vi "Flatten To String.vi"(8 "error in (no error)":errorcluster, 10 "Variant":variant, 11 "JSON Serializer in":refnum<class "JSON Serializer.lvclass">) -> (0 "error out":errorcluster, 2 "String":string, 3 "JSON Serializer out":refnum<class "JSON Serializer.lvclass">)   [LabVIEW 2017, in "JKI JSON Serialization.lvlib" / "JSON Serializer.lvclass"]
doc: "Converts <b>Variant</b> to JSON formatted <b>String</b>."
uses:
  JSON Serializer.lvclass
  JSON Serializer.lvclass/JSON Serializer.ctl
  <vilib>/Utility/error.llb/whitespace.ctl
  <vilib>/Utility/VariantDataType/VariantType.lvlib
  JKI JSON Serialization.lvlib
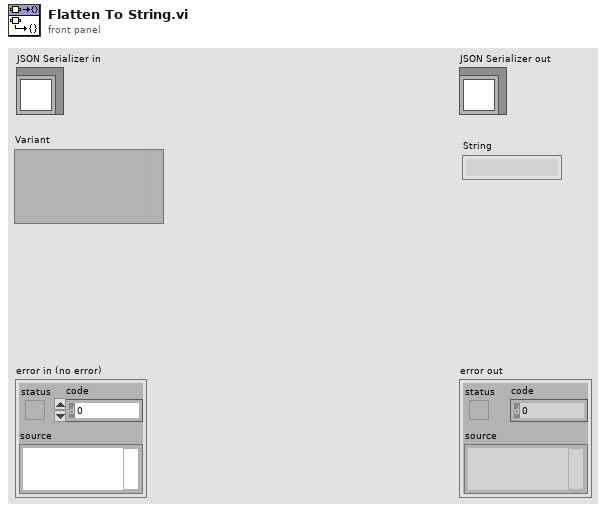
[diagram p1: front panel]
types:
  T1 = typedef "VariantType.lvlib/Type.ctl" = enum8{"Invalid Type", "Void", "I8", "I16", "I32", "I64", "U8", "U16", "U32", "U64", "Single Float", "Double Float", "Extended Float", "Single Complex", "Double Complex", "Extended Complex", "Enum U8", "Enum U16", "Enum U32", "Enum U64", "Single Float With Unit", "Double Float With Unit", "Extended Float With Unit", "Single Complex with Unit", "Double Complex with Unit", "Extended Complex with Unit", "Boolean", "String", "Path", "Picture", "Tag", "Array", "Cluster", "Variant", "LV Variant", "Waveform", "Timestamp", "Digital Waveform", "Digital Data", "ExpressData", "Refnum", "External Data", "VI", "Poly VI", "LabVIEW Class Instance", "Fixed Point"}
  T2 = typedef "whitespace.ctl" = u16
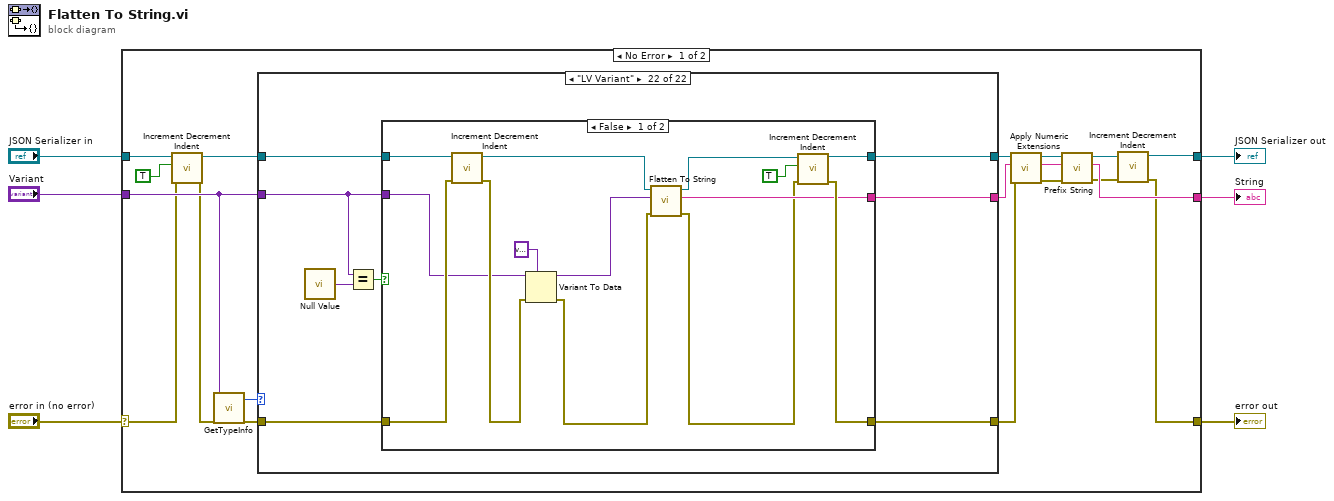
[diagram p0: block diagram]
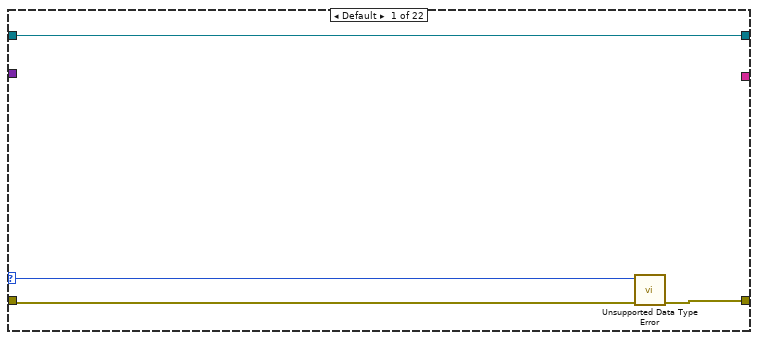
[diagram p2: hidden frame]
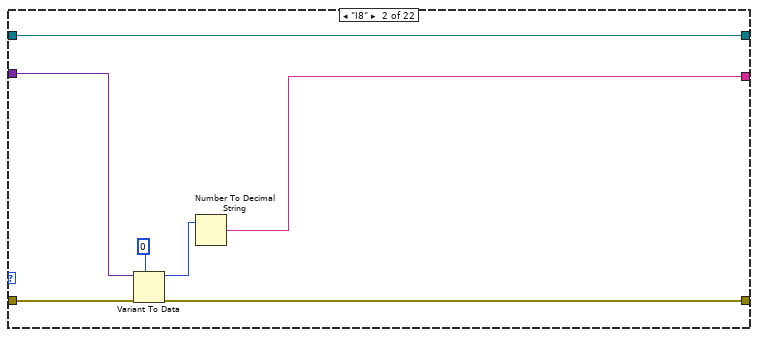
[diagram p3: hidden frame]
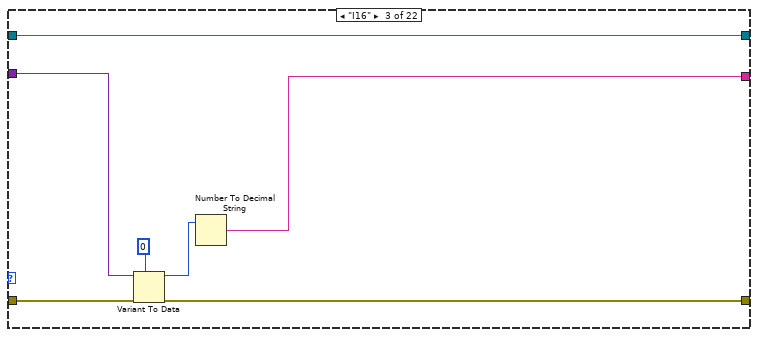
[diagram p4: hidden frame]
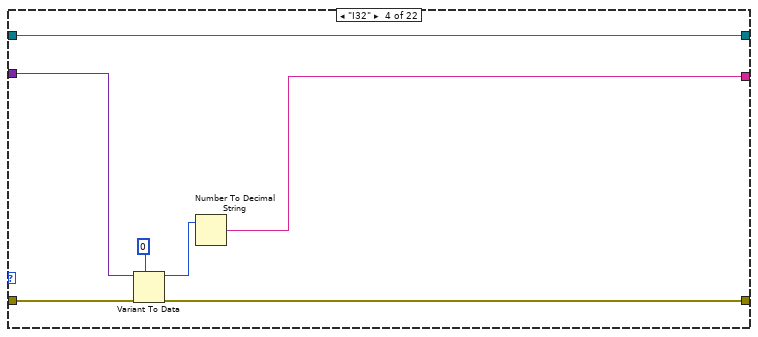
[diagram p5: hidden frame]
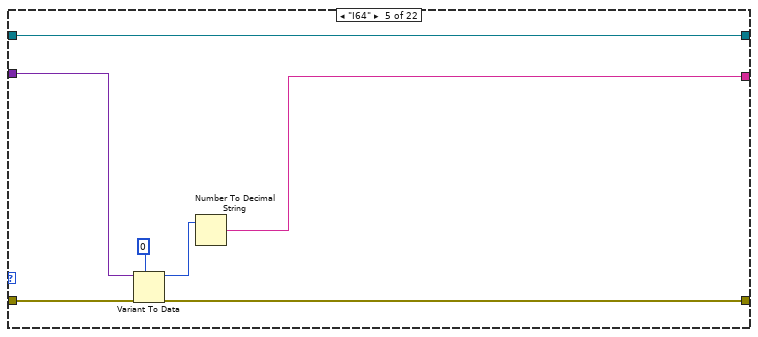
[diagram p6: hidden frame]
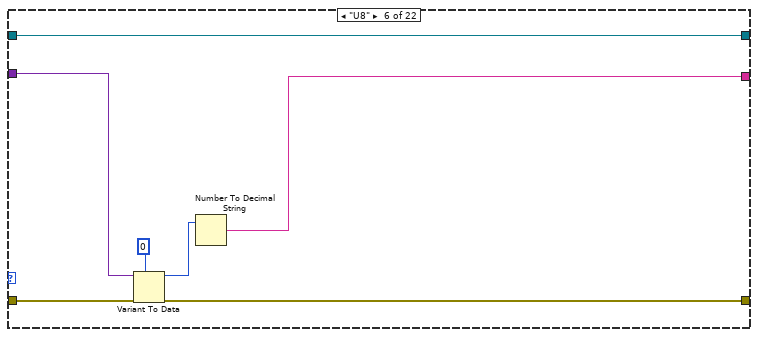
[diagram p7: hidden frame]
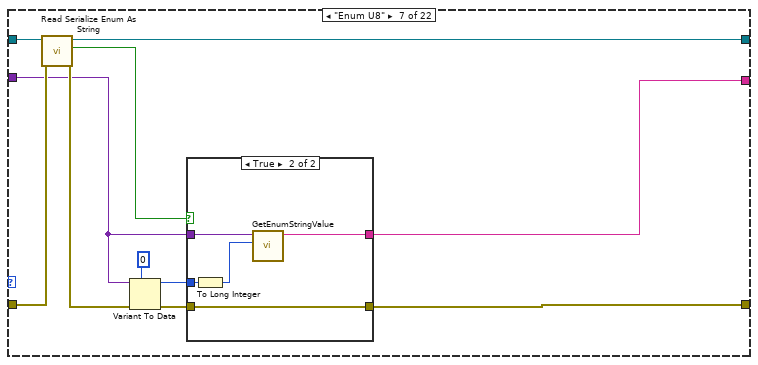
[diagram p8: hidden frame]
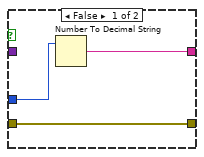
[diagram p9: hidden frame]
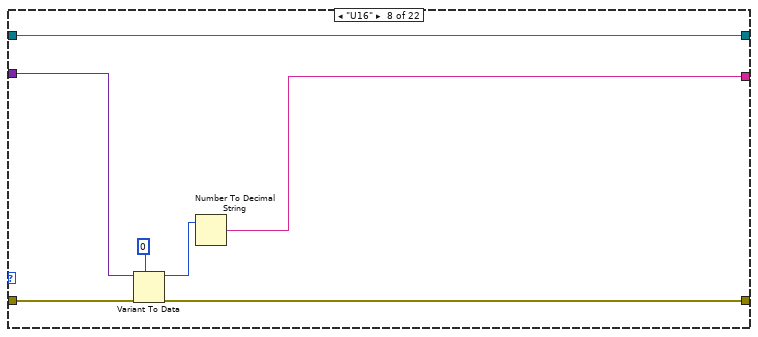
[diagram p10: hidden frame]
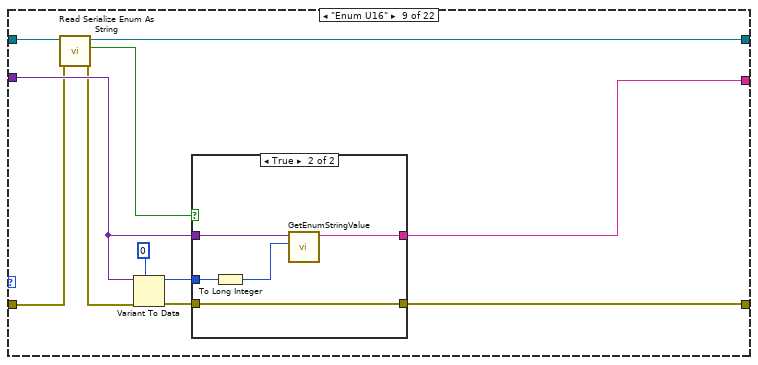
[diagram p11: hidden frame]
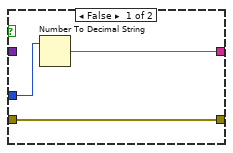
[diagram p12: hidden frame]
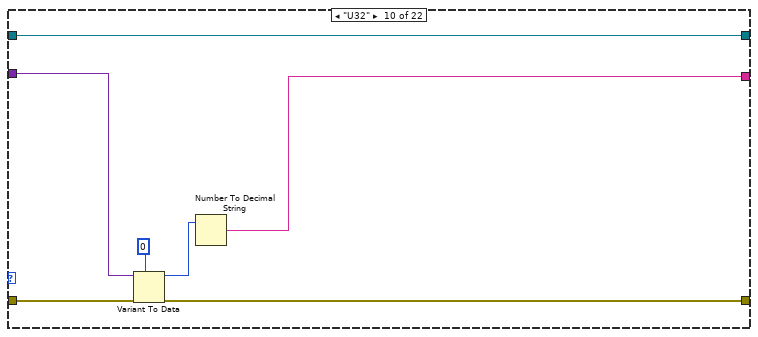
[diagram p13: hidden frame]
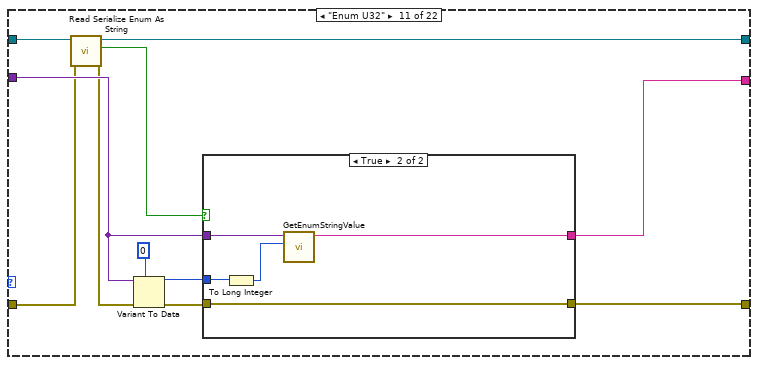
[diagram p14: hidden frame]
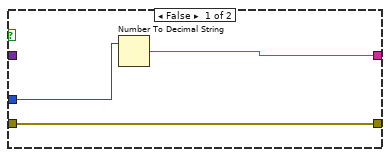
[diagram p15: hidden frame]
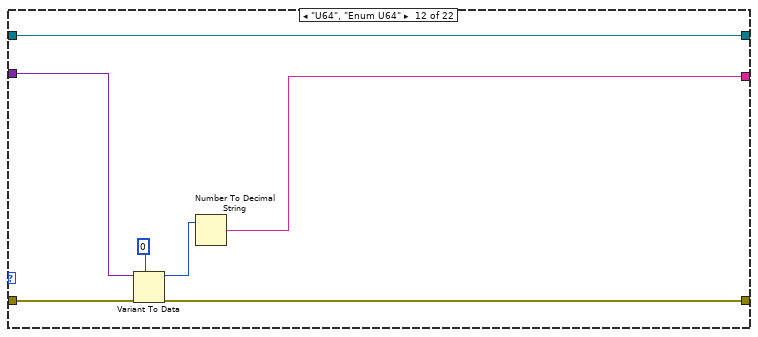
[diagram p16: hidden frame]
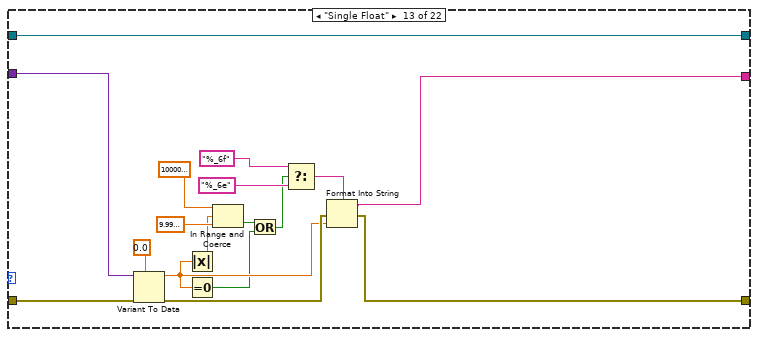
[diagram p17: hidden frame]
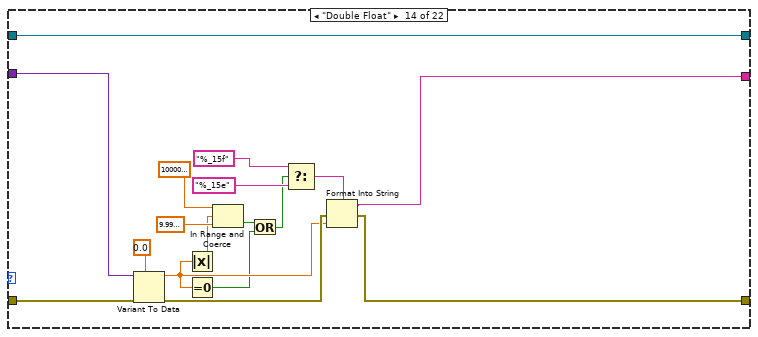
[diagram p18: hidden frame]
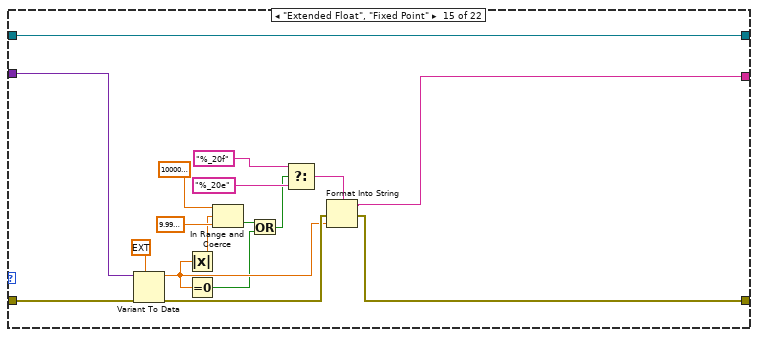
[diagram p19: hidden frame]
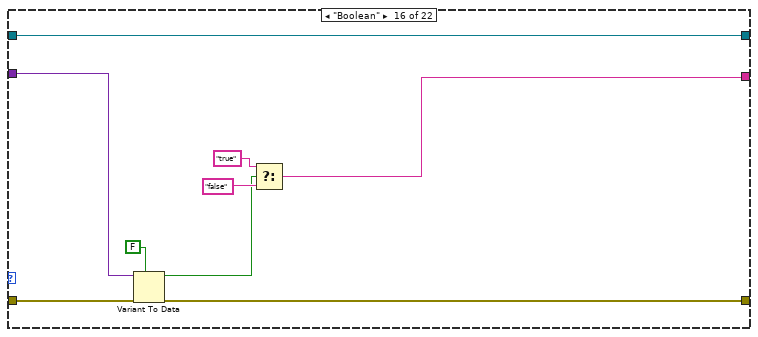
[diagram p20: hidden frame]
diagram:
  n1 = case shown="No Error" "error in (no error)" {
    selector: "error in (no error)" -> [w18 w436]
    tunnel: [w7 w436] -> w5
    tunnel: [w9 w435] -> w3
    tunnel: "JSON Serializer in" -> [w20 w435]
    tunnel: "Variant" -> [w23 _]
    tunnel: [w12 _] -> w1
    frame No Error {
      n2 = call "Increment Decrement Indent.vi"("error in (no error)"=w18, "Increment"=TRUE, "JSON Serializer in"=w20) -> ("error out"=w17:errorcluster, "JSON Serializer out"=w19:refnum<class "JSON Serializer.lvclass">)  [unwired: 7 in]
      n3 = call <vilib>:"GetTypeInfo.vi"("error in (no error)"=w17, "Variant"=w23) -> ("error out"=w24:errorcluster, "Type Enum"=w25:T1)  [unwired: 5 in, 3 out]
      n4 = case shown="\"LV Variant\"" w25 {
        selector: w25 -> [w26 _ _ _ _ _ _ _ _ _ _ _ _ _ _ _ w203 w250 _ _ _ _]
        tunnel: w19 -> [w29 w36 w43 w50 w57 w64 w74 w90 w95 w116 w125 w142 w159 w176 w193 w202 w208 w248 w275 w323 w358 w414]
        tunnel: [w29 w36 w43 w50 w57 w64 w73 w90 w94 w116 w124 w142 w159 w176 w193 w202 w208 w247 w274 w321 w361 w417] -> w15
        tunnel: [w28 w30 w37 w44 w51 w58 w65 w84 w98 w110 w122 w136 w154 w171 w188 w194 w205 w251 w273 w320 w360 w416] -> w22
        tunnel: w24 -> [w27 w35 w42 w49 w56 w63 w72 w89 w93 w115 w118 w141 w158 w175 w192 w201 w207 w249 w271 w324 w362 w413]
        tunnel: [_ w31 w38 w45 w52 w59 w75 w85 w97 w111 w123 w137 w148 w165 w182 w196 w204 w245 w272 w319 w359 w415] -> w21
        tunnel: w23 -> [_ w34 w41 w48 w55 w62 w67 w88 w96 w114 w119 w140 w157 w174 w191 w200 w206 w243 w269 w322 w363 w411]
        frame Default {
          n5 = call "Unsupported Data Type Error.vi"("error in (no error)"=w27, "Type Enum"=w26) -> ("error out"=w28:errorcluster)  [unwired: 9 in]
        }
        frame "I8" {
          n6 = Variant To Data(error in=w35, type=i8 0, Variant=w34) -> (data=w32:i8, error out=w30:errorcluster)
          n7 = Number To Decimal String(number=w32) -> (decimal integer string=w31:string)  [unwired: 1 in]
        }
        frame "I16" {
          n8 = Variant To Data(error in=w42, type=i16 0, Variant=w41) -> (data=w39:i16, error out=w37:errorcluster)
          n9 = Number To Decimal String(number=w39) -> (decimal integer string=w38:string)  [unwired: 1 in]
        }
        frame "I32" {
          n10 = Variant To Data(error in=w49, type=0, Variant=w48) -> (data=w46:i32, error out=w44:errorcluster)
          n11 = Number To Decimal String(number=w46) -> (decimal integer string=w45:string)  [unwired: 1 in]
        }
        frame "I64" {
          n12 = Variant To Data(error in=w56, type=i64 0, Variant=w55) -> (data=w53:i64, error out=w51:errorcluster)
          n13 = Number To Decimal String(number=w53) -> (decimal integer string=w52:string)  [unwired: 1 in]
        }
        frame "U8" {
          n14 = Variant To Data(error in=w63, type=u8 0, Variant=w62) -> (data=w60:u8, error out=w58:errorcluster)
          n15 = Number To Decimal String(number=w60) -> (decimal integer string=w59:string)  [unwired: 1 in]
        }
        frame "Enum U8" {
          n16 = call-dynamic "Read Serialize Enum As String.vi"("error in (no error)"=w72, "JSON Serializer in"=w74) -> ("error out"=w71:errorcluster, "Enums As String?"=w68:bool, "JSON Serializer out"=w73:refnum<class "JSON Serializer.lvclass">)  [unwired: 7 in]
          n17 = Variant To Data(error in=w71, type=u8 0, Variant=w67) -> (data=w69:u8, error out=w66:errorcluster)
          n18 = case shown="True" w68 {
            tunnel: [w78 w79] -> w75
            tunnel: w69 -> [w77 w81]
            tunnel: w67 -> [_ w82]
            tunnel: w66 -> [w76 w83]
            tunnel: [w76 w83] -> w65
            frame False {
              n19 = Number To Decimal String(number=w77) -> (decimal integer string=w78:string)  [unwired: 1 in]
            }
            frame True {
              n20 = To Long Integer(number=w81) -> (32bit integer=w80:i32)
              n21 = call "GetEnumStringValue.vi"("Index"=w80, "Enum Variant"=w82) -> ("string"=w79:string)  [unwired: 9 in]
            }
          }
        }
        frame "U16" {
          n22 = Variant To Data(error in=w89, type=u16 0, Variant=w88) -> (data=w86:u16, error out=w84:errorcluster)
          n23 = Number To Decimal String(number=w86) -> (decimal integer string=w85:string)  [unwired: 1 in]
        }
        frame "Enum U16" {
          n24 = call-dynamic "Read Serialize Enum As String.vi"("error in (no error)"=w93, "JSON Serializer in"=w95) -> ("error out"=w92:errorcluster, "Enums As String?"=w91:bool, "JSON Serializer out"=w94:refnum<class "JSON Serializer.lvclass">)  [unwired: 7 in]
          n25 = Variant To Data(error in=w92, type=u16 0, Variant=w96) -> (data=w100:u16, error out=w99:errorcluster)
          n26 = case shown="True" w91 {
            tunnel: [w104 w105] -> w97
            tunnel: w100 -> [w103 w107]
            tunnel: w96 -> [_ w108]
            tunnel: w99 -> [w102 w106]
            tunnel: [w102 w106] -> w98
            frame False {
              n27 = Number To Decimal String(number=w103) -> (decimal integer string=w104:string)  [unwired: 1 in]
            }
            frame True {
              n28 = To Long Integer(number=w107) -> (32bit integer=w109:i32)
              n29 = call "GetEnumStringValue.vi"("Index"=w109, "Enum Variant"=w108) -> ("string"=w105:string)  [unwired: 9 in]
            }
          }
        }
        frame "U32" {
          n30 = Variant To Data(error in=w115, type=u32 0, Variant=w114) -> (data=w112:u32, error out=w110:errorcluster)
          n31 = Number To Decimal String(number=w112) -> (decimal integer string=w111:string)  [unwired: 1 in]
        }
        frame "Enum U32" {
          n32 = call-dynamic "Read Serialize Enum As String.vi"("error in (no error)"=w118, "JSON Serializer in"=w125) -> ("error out"=w117:errorcluster, "Enums As String?"=w126:bool, "JSON Serializer out"=w124:refnum<class "JSON Serializer.lvclass">)  [unwired: 7 in]
          n33 = Variant To Data(error in=w117, type=u32 0, Variant=w119) -> (data=w120:u32, error out=w121:errorcluster)
          n34 = case shown="True" w126 {
            tunnel: [w130 w131] -> w123
            tunnel: w120 -> [w129 w132]
            tunnel: w119 -> [_ w133]
            tunnel: w121 -> [w128 w135]
            tunnel: [w128 w135] -> w122
            frame False {
              n35 = Number To Decimal String(number=w129) -> (decimal integer string=w130:string)  [unwired: 1 in]
            }
            frame True {
              n36 = To Long Integer(number=w132) -> (32bit integer=w134:i32)
              n37 = call "GetEnumStringValue.vi"("Index"=w134, "Enum Variant"=w133) -> ("string"=w131:string)  [unwired: 9 in]
            }
          }
        }
        frame "U64", "Enum U64" {
          n38 = Variant To Data(error in=w141, type=u64 0, Variant=w140) -> (data=w138:u64, error out=w136:errorcluster)
          n39 = Number To Decimal String(number=w138) -> (decimal integer string=w137:string)  [unwired: 1 in]
        }
        frame "Single Float" {
          n40 = Variant To Data(error in=w158, type=sgl 0.0, Variant=w157) -> (data=w146:sgl, error out=w155:errorcluster)
          n41 = Absolute Value(x=w146) -> (abs(x)=w147:sgl)
          n42 = Equal To 0?(x=w146) -> (x = 0?=w145:bool)
          n43 = In Range and Coerce(upper limit=sgl 1000000.0, x=w147, lower limit=sgl 0.0001 ("upper limit")) -> (In Range?=w144:bool)  [unwired: 1 out]
          n44 = Or(x=w144, y=w145) -> (x .or. y?=w143:bool)
          n45 = Select(t="%_6f" ("format string"), s=w143, f="%_6e" ("format string")) -> (s? t:f=w149:string)
          n46 = Format Into String(format string=w149, error in=w155, w146) -> (resulting string=w148:string, error out=w154:errorcluster)  [unwired: 1 in]
        }
        frame "Double Float" {
          n47 = Variant To Data(error in=w175, type=0.0, Variant=w174) -> (data=w163:dbl, error out=w172:errorcluster)
          n48 = Absolute Value(x=w163) -> (abs(x)=w164:dbl)
          n49 = Equal To 0?(x=w163) -> (x = 0?=w162:bool)
          n50 = In Range and Coerce(upper limit=sgl 1000000.0, x=w164, lower limit=sgl 0.0001 ("upper limit")) -> (In Range?=w161:bool)  [unwired: 1 out]
          n51 = Or(x=w161, y=w162) -> (x .or. y?=w160:bool)
          n52 = Select(t="%_15f" ("format string"), s=w160, f="%_15e" ("format string")) -> (s? t:f=w166:string)
          n53 = Format Into String(format string=w166, error in=w172, w163) -> (resulting string=w165:string, error out=w171:errorcluster)  [unwired: 1 in]
        }
        frame "Extended Float", "Fixed Point" {
          n54 = Variant To Data(error in=w192, type=ext 0.0, Variant=w191) -> (data=w180:ext, error out=w189:errorcluster)
          n55 = Absolute Value(x=w180) -> (abs(x)=w181:ext)
          n56 = Equal To 0?(x=w180) -> (x = 0?=w179:bool)
          n57 = In Range and Coerce(upper limit=sgl 1000000.0, x=w181, lower limit=sgl 0.0001 ("upper limit")) -> (In Range?=w178:bool)  [unwired: 1 out]
          n58 = Or(x=w178, y=w179) -> (x .or. y?=w177:bool)
          n59 = Select(t="%_20f" ("format string"), s=w177, f="%_20e" ("format string")) -> (s? t:f=w183:string)
          n60 = Format Into String(format string=w183, error in=w189, w180) -> (resulting string=w182:string, error out=w188:errorcluster)  [unwired: 1 in]
        }
        frame "Boolean" {
          n61 = Variant To Data(error in=w201, type=FALSE, Variant=w200) -> (data=w195:bool, error out=w194:errorcluster)
          n62 = Select(t="true" ("format string"), s=w195, f="false" ("format string")) -> (s? t:f=w196:string)
        }
        frame "String", "Path" {
          n63 = case shown="\"Path\"" w203 {
            tunnel: w207 -> [w216 w242]
            tunnel: w206 -> [w215 w241]
            tunnel: [w214 w237] -> w205
            tunnel: [w213 w231] -> w204
            frame "Path" {
              n64 = Variant To Data(error in=w216, type=path "", Variant=w215) -> (data=w209:path, error out=w211:errorcluster)
              n65 = Not A Number/Path/Refnum?(number/path/refnum=w209) -> (NaN/Path/Refnum?=w210:bool)
              n66 = case shown="True" w210 {
                tunnel: [w225 w229] -> w214
                tunnel: [w219 "null" ("JSON string")] -> w213
                tunnel: w211 -> [w217 w229]
                tunnel: w209 -> [w218 _]
                frame False {
                  n67 = Path To String(path=w218) -> (string=w226:string)
                  n68 = Build Array(w226) -> (w227:string[])
                  n69 = Flatten To JSON(anything=w227, error in (no error)=w217) -> (JSON string=w223:string, 11:w225:errorcluster)  [unwired: 1 in]
                  n70 = String Length(string=w223) -> (length=w222:i32)
                  n71 = Subtract(x=w222, y=2) -> (x-y=w220:i32)
                  n72 = String Subset(string=w223, offset (0)=1, length (rest)=w220) -> (substring=w219:string)
                }
                frame True {
                }
              }
            }
            frame "String", Default {
              n73 = Variant To Data(error in=w242, type="", Variant=w241) -> (data=w239:string, error out=w238:errorcluster)
              n74 = Build Array(w239) -> (w240:string[])
              n75 = Flatten To JSON(anything=w240, error in (no error)=w238) -> (JSON string=w235:string, 11:w237:errorcluster)  [unwired: 1 in]
              n76 = String Length(string=w235) -> (length=w234:i32)
              n77 = Subtract(x=w234, y=2) -> (x-y=w232:i32)
              n78 = String Subset(string=w235, offset (0)=1, length (rest)=w232) -> (substring=w231:string)
            }
          }
        }
        frame "Timestamp" {
          n79 = Unbundle By Name(w248) -> ("timestamps"=w246:bool, "universal time"=w244:bool)
          n80 = case shown="True" w246 {
            tunnel: [w255 w256] -> w251
            tunnel: w250 -> [w254 _]
            tunnel: w249 -> [w253 w266]
            tunnel: w248 -> [w252 w267]
            tunnel: [w252 w267] -> w247
            tunnel: [_ w258] -> w245
            tunnel: w244 -> [_ w261]
            tunnel: w243 -> [_ w265]
            frame False {
              n81 = call "Unsupported Data Type Error.vi"("error in (no error)"=w253, "Type Enum"=w254) -> ("error out"=w255:errorcluster)  [unwired: 9 in]
            }
            frame True {
              n82 = Variant To Data(error in=w266, type=timestamp(0 s since 1904-01-01), Variant=w265) -> (data=w264:timestamp, error out=w262:errorcluster)
              n83 = call "Timestamp To ISO String.vi"("error in (no error)"=w262, "Universal time (F)"=w261, "Timestamp"=w264) -> ("error out"=w257:errorcluster, "ISO Timestamp String"=w259:string)  [unwired: 7 in]
              n84 = Format Into String(format string="\"%s\"", error in=w257, w259) -> (resulting string=w258:string, error out=w256:errorcluster)  [unwired: 1 in]
            }
          }
        }
        frame "Array" {
          n85 = call <vilib>:"GetArrayInfo.vi"("error in (no error)"=w271, "Variant"=w269) -> ("error out"=w270:errorcluster, "NDims"=w268:i32)  [unwired: 6 in, 2 out]
          n86 = case shown="2.." w268 {
            tunnel: w275 -> [w276 w292 w312]
            tunnel: [w276 w289 w310] -> w274
            tunnel: [w279 w287 w308] -> w273
            tunnel: [_ w286 w307] -> w272
            tunnel: w270 -> [w277 w282 w302]
            tunnel: w269 -> [_ w281 w303]
            frame 0, Default {
              n87 = call <vilib>:"Error Cluster From Error Code.vi"("error in (no error)"=w277, "error message (\"\")"="Flattening failed. Zero or negative dimensional arrays not supported." ("error message (\"\")"), "error code (0)"=1) -> ("error out"=w279:errorcluster)  [unwired: 6 in]
            }
            frame 1 {
              n88 = call <userlib>:"Array to Array of VData__ogtk.vi"("error in (no error)"=w282, "MultiD Array"=w281) -> ("error out"=w291:errorcluster, "1D Array of Variants"=w293:variant[])  [unwired: 8 in]
              n89 = for {
                tunnel: w293 -> [w299] mode=indexing
                shift-right: [w297] -> w290
                shift-left: w292 -> [w298]
                tunnel: [w296] -> w285 mode=indexing
                shift-right: [w295] -> w288
                shift-left: w291 -> [w294]
                n90 = call-dynamic "Flatten To String.vi"("error in (no error)"=w294, "Variant"=w299, "JSON Serializer in"=w298) -> ("error out"=w295:errorcluster, "String"=w296:string, "JSON Serializer out"=w297:refnum<class "JSON Serializer.lvclass">)  [unwired: 6 in]
              }
              n91 = call "Prefix Array.vi"("End Symbol"="]", "Start Symbol"="[", "error in (no error)"=w288, "Array"=w285, "JSON Serializer in"=w290) -> ("error out"=w287:errorcluster, "String"=w286:string, "JSON Serializer out"=w289:refnum<class "JSON Serializer.lvclass">)  [unwired: 4 in]
            }
            frame 2.. {
              n92 = call "MultiD Array to 1D Array of VArrays.vi"("error in (no error)"=w302, "MultiD Array"=w303) -> ("error out"=w301:errorcluster, "Array of VArrays"=w300:variant[])  [unwired: 8 in]
              n93 = for {
                tunnel: w300 -> [w318] mode=indexing
                shift-right: [w316] -> w311
                shift-left: w312 -> [w317]
                tunnel: [w315] -> w306 mode=indexing
                shift-right: [w314] -> w309
                shift-left: w301 -> [w313]
                n94 = call-dynamic "Flatten To String.vi"("error in (no error)"=w313, "Variant"=w318, "JSON Serializer in"=w317) -> ("error out"=w314:errorcluster, "String"=w315:string, "JSON Serializer out"=w316:refnum<class "JSON Serializer.lvclass">)  [unwired: 6 in]
              }
              n95 = call "Prefix Array.vi"("End Symbol"="]", "Start Symbol"="[", "error in (no error)"=w309, "Array"=w306, "JSON Serializer in"=w311) -> ("error out"=w308:errorcluster, "String"=w307:string, "JSON Serializer out"=w310:refnum<class "JSON Serializer.lvclass">)  [unwired: 4 in]
            }
          }
        }
        frame "Void" {
          # "Void varients are used as run-time defineable objects, with key-value pairs stored as variant attributes.\nIf no attributes are defined, returns empty object \"{}\""
          n96 = Get Variant Attribute(Variant=w322, error in=w324) -> (names=w332:string[], values=w333:variant[], error out=w331:errorcluster)  [unwired: 2 in, 1 out]
          n97 = Unbundle By Name(w323) -> ("multiline?"=w325:bool)
          n98 = for {
            tunnel: w333 -> [w339] mode=indexing
            shift-right: [w334] -> w330
            shift-left: w323 -> [w345]
            tunnel: [w344] -> w326 mode=indexing
            shift-right: [w349] -> w329
            shift-left: w331 -> [w348]
            tunnel: w325 -> [w340]
            tunnel: w332 -> [w338] mode=indexing
            n99 = To Variant(anything=w338) -> (Variant=w337:variant)
            n100 = call-dynamic "Flatten To String.vi"("error in (no error)"=w348, "Variant"=w339, "JSON Serializer in"=w345) -> ("error out"=w347:errorcluster, "String"=w342:string, "JSON Serializer out"=w335:refnum<class "JSON Serializer.lvclass">)  [unwired: 6 in]
            n101 = case shown="True" w340 {
              tunnel: w342 -> [w350 w353]
              tunnel: [w350 w351] -> w341
              frame False {
              }
              frame True {
                w352 = T2 1 items=["both", "start of string", "end of string"] ("location (both)")
                n102 = call <vilib>:"Trim Whitespace.vi"("string"=w353, "location (both)"=w352) -> ("trimmed string"=w351:string)
              }
            }
            n103 = call-dynamic "Flatten To String.vi"("error in (no error)"=w347, "Variant"=w337, "JSON Serializer in"=w335) -> ("error out"=w346:errorcluster, "String"=w336:string, "JSON Serializer out"=w334:refnum<class "JSON Serializer.lvclass">)  [unwired: 6 in]
            n104 = Format Into String(format string="%s:%s", error in=w346, w336, w341) -> (resulting string=w344:string, error out=w349:errorcluster)  [unwired: 1 in]
          }
          n105 = call "Prefix Array.vi"("End Symbol"="}", "Start Symbol"="{", "error in (no error)"=w329, "Array"=w326, "JSON Serializer in"=w330) -> ("error out"=w320:errorcluster, "String"=w319:string, "JSON Serializer out"=w321:refnum<class "JSON Serializer.lvclass">)  [unwired: 4 in]
        }
        frame "Cluster" {
          n106 = call "Cluster Info.vi"("error in (no error)"=w362, "Cluster Variant"=w363) -> ("error out"=w357:errorcluster, "Name"=w354:string, "Treat As Array"=w355:bool, "Cluster Elements"=w356:variant[])  [unwired: 6 in]
          n107 = case shown="False" w355 {
            tunnel: [w374 w402] -> w361
            tunnel: [w372 w399] -> w360
            tunnel: [w368 w405] -> w359
            tunnel: w358 -> [w367 w404]
            tunnel: w357 -> [w365 w397]
            tunnel: w356 -> [w364 w409]
            tunnel: w354 -> [_ w408]
            frame False {
              # "Treat cluster as an object"
              n108 = Unbundle By Name(w367) -> ("multiline?"=w366:bool)
              n109 = for {
                tunnel: w364 -> [w376] mode=indexing
                shift-right: [w386] -> w375
                shift-left: w367 -> [w391]
                tunnel: [w388] -> w369 mode=indexing
                shift-right: [w389] -> w373
                shift-left: w365 -> [w379]
                tunnel: w366 -> [w380]
                n110 = call "Variant Metadata.vi"("error in (no error)"=w379, "Variant"=w376) -> ("error out"=w378:errorcluster, "Name"=w377:string)  [unwired: 7 in, 1 out]
                n111 = call-dynamic "Flatten To String.vi"("error in (no error)"=w378, "Variant"=w376, "JSON Serializer in"=w391) -> ("error out"=w390:errorcluster, "String"=w382:string, "JSON Serializer out"=w387:refnum<class "JSON Serializer.lvclass">)  [unwired: 6 in]
                n112 = case shown="True" w380 {
                  tunnel: w382 -> [w392 w395]
                  tunnel: [w392 w393] -> w381
                  frame False {
                  }
                  frame True {
                    w394 = T2 1 items=["both", "start of string", "end of string"] ("location (both)")
                    n113 = call <vilib>:"Trim Whitespace.vi"("string"=w395, "location (both)"=w394) -> ("trimmed string"=w393:string)
                  }
                }
                n114 = call-dynamic "Flatten To String.vi"("error in (no error)"=w390, "Variant"=w377, "JSON Serializer in"=w387) -> ("error out"=w385:errorcluster, "String"=w384:string, "JSON Serializer out"=w386:refnum<class "JSON Serializer.lvclass">)  [unwired: 6 in]
                n115 = Format Into String(format string="%s:%s", error in=w385, w384, w381) -> (resulting string=w388:string, error out=w389:errorcluster)  [unwired: 1 in]
              }
              n116 = call "Prefix Array.vi"("End Symbol"="}", "Start Symbol"="{", "error in (no error)"=w373, "Array"=w369, "JSON Serializer in"=w375) -> ("error out"=w372:errorcluster, "String"=w368:string, "JSON Serializer out"=w374:refnum<class "JSON Serializer.lvclass">)  [unwired: 4 in]
            }
            frame True {
              # "Treat cluster as an ordered array"
              n117 = call "Increment Decrement Indent.vi"("error in (no error)"=w397, "JSON Serializer in"=w404) -> ("error out"=w396:errorcluster, "JSON Serializer out"=w403:refnum<class "JSON Serializer.lvclass">)  [unwired: 8 in]
              n118 = call <userlib>:"Set Data Name__ogtk.vi"("error in (no error)"=w396, "Data Name"=w408, "Data"=w409) -> ("error out"=w407:errorcluster, "Renamed Data"=w406:variant)  [unwired: 7 in]
              n119 = call-dynamic "Flatten To String.vi"("error in (no error)"=w407, "Variant"=w406, "JSON Serializer in"=w403) -> ("error out"=w400:errorcluster, "String"=w405:string, "JSON Serializer out"=w401:refnum<class "JSON Serializer.lvclass">)  [unwired: 6 in]
              n120 = call "Increment Decrement Indent.vi"("error in (no error)"=w400, "Increment"=TRUE, "JSON Serializer in"=w401) -> ("error out"=w399:errorcluster, "JSON Serializer out"=w402:refnum<class "JSON Serializer.lvclass">)  [unwired: 7 in]
            }
          }
        }
        frame "LV Variant" {
          n121 = call "Null Value.vi"() -> ("Null"=w410:variant)
          n122 = Equal?(x=w411, y=w410) -> (x = y?=w412:bool)
          n123 = case shown="False" w412 {
            tunnel: [w431 w434] -> w417
            tunnel: [w430 w433] -> w416
            tunnel: [w429 "null" ("String")] -> w415
            tunnel: w414 -> [w428 w434]
            tunnel: w413 -> [w421 w433]
            tunnel: w411 -> [w418 _]
            frame False {
              n124 = call "Increment Decrement Indent.vi"("error in (no error)"=w421, "JSON Serializer in"=w428) -> ("error out"=w423:errorcluster, "JSON Serializer out"=w427:refnum<class "JSON Serializer.lvclass">)  [unwired: 8 in]
              n125 = Variant To Data(error in=w423, type=variant ("variant"), Variant=w418) -> (data=w420:variant, error out=w419:errorcluster)
              n126 = call-dynamic "Flatten To String.vi"("error in (no error)"=w419, "Variant"=w420, "JSON Serializer in"=w427) -> ("error out"=w425:errorcluster, "String"=w429:string, "JSON Serializer out"=w426:refnum<class "JSON Serializer.lvclass">)  [unwired: 6 in]
              n127 = call "Increment Decrement Indent.vi"("error in (no error)"=w425, "Increment"=TRUE, "JSON Serializer in"=w426) -> ("error out"=w430:errorcluster, "JSON Serializer out"=w431:refnum<class "JSON Serializer.lvclass">)  [unwired: 7 in]
            }
            frame True {
            }
          }
        }
      }
      n128 = call "Apply Numeric Extensions.vi"("error in (no error)"=w22, "JSON string in"=w21, "JSON Serializer in"=w15) -> ("error out"=w8:errorcluster, "JSON string out"=w13:string, "JSON Serializer out"=w14:refnum<class "JSON Serializer.lvclass">)  [unwired: 6 in]
      n129 = call "Prefix String.vi"("error in (no error)"=w8, "Input String"=w13, "JSON Serializer in"=w14) -> ("error out"=w10:errorcluster, "Output String"=w12:string, "JSON Serializer out"=w11:refnum<class "JSON Serializer.lvclass">)  [unwired: 6 in]
      n130 = call "Increment Decrement Indent.vi"("error in (no error)"=w10, "JSON Serializer in"=w11) -> ("error out"=w7:errorcluster, "JSON Serializer out"=w9:refnum<class "JSON Serializer.lvclass">)  [unwired: 8 in]
    }
    frame Error {
    }
  }
  "error out" <- w5
  "JSON Serializer out" <- w3
  "String" <- w1
